vi "Invalid for Named.vi"(8 "error in (no error)":errorcluster, 11 "NamedPackage in":refnum<class "NamedPackage.lvclass">) -> (0 "error out":errorcluster, 3 "NamedPackage out":refnum<class "NamedPackage.lvclass">)   [LabVIEW 2020, in "GPack.lvlib" / "NamedPackage.lvclass"]
uses:
  NamedPackage.lvclass
  NamedPackage.lvclass/NamedPackage.ctl
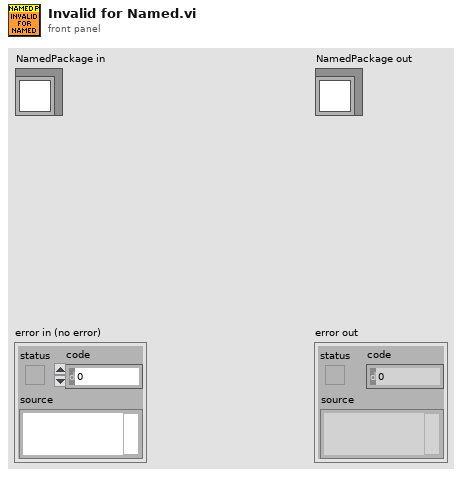
[diagram p1: front panel]
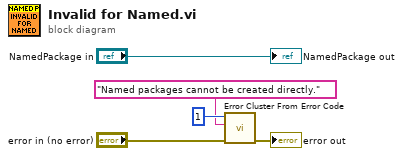
[diagram p0: block diagram]
diagram:
  n1 = call <vilib>:"Error Cluster From Error Code.vi"("error in (no error)"="error in (no error)", "error message (\"\")"="Named packages cannot be created directly.", "error code (0)"=1) -> ("error out"=→"error out":errorcluster)  [unwired: 6 in]
  "NamedPackage out" <- "NamedPackage in"
